vi "Match first tags.vi"(9 "Hyperlink":string, 11 "Text":string) -> (1 "Array":T2(array[cluster]), 3 "Find tag ?":bool)   [LabVIEW 2019, in "Exaprom PDF.lvlib"]
doc: "Version 1.0\nDeveloped by Jean-Marc Simard\nCopyright © 2010, Exaprom Inc.\nAll rights reserved.\nLicense: BSD"
uses:
  Controls/Text Controls/Text type.ctl
  Exaprom PDF.lvlib
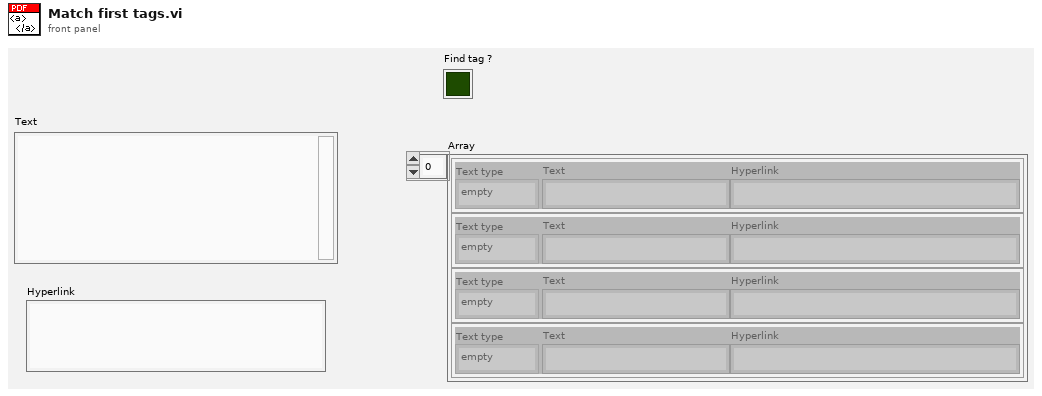
[diagram p1: front panel]
types:
  T1 = typedef "Exaprom PDF.lvlib/Text type.ctl" = enum16{"empty", "Text", "Hyperlink"}
  T2 = cluster{"Text type":T1, "Text":string, "Hyperlink":string}[]
  T3 = cluster{"Text type":T1, "Text type":T1, "Text type":T1}
  T4 = cluster{"Text type":T1, "Text":string, "Hyperlink":string}
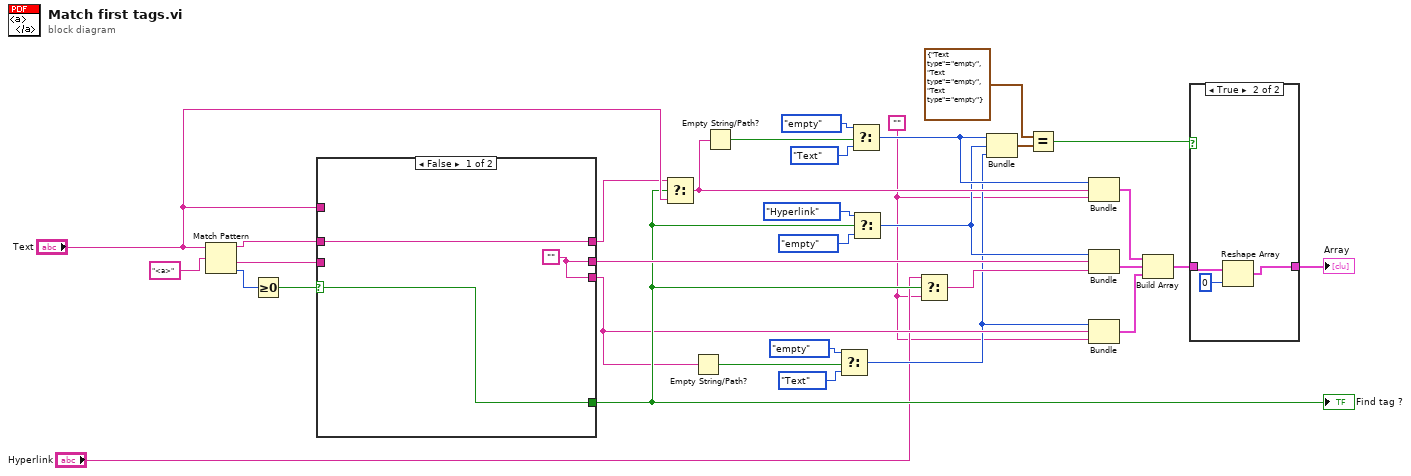
[diagram p0: block diagram]
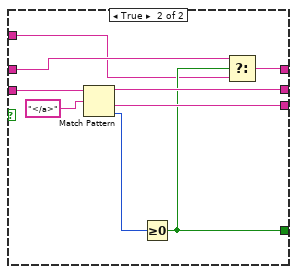
[diagram p3: hidden frame]
diagram:
  w1 = ""
  n1 = Match Pattern(string="Text", regular expression="<a>") -> (before substring=w29:string, after substring=w28:string, offset past match=w32:i32)  [unwired: 2 out]
  n2 = Greater Or Equal To 0?(x=w32) -> (x >= 0?=w31:bool)
  n3 = case shown="False" w31 {
    selector: w31 -> [w34 _]
    tunnel: w29 -> [w36 w38]
    tunnel: [w36 w40] -> w22
    tunnel: w28 -> [_ w45]
    tunnel: [w35 w43] -> w27
    tunnel: [w35 w42] -> w11
    tunnel: [w34 w39] -> w16
    tunnel: "Text" -> [_ w37]
    frame False {
      w35 = ""
    }
    frame True {
      n4 = Match Pattern(string=w45, regular expression="</a>") -> (before substring=w43:string, after substring=w42:string, offset past match=w41:i32)  [unwired: 2 out]
      n5 = Greater Or Equal To 0?(x=w41) -> (x >= 0?=w39:bool)
      n6 = Select(t=w38, s=w39, f=w37) -> (s? t:f=w40:string)
    }
  }
  "Find tag ?" <- w16
  n7 = Select(t=w22, s=w16, f="Text") -> (s? t:f=w15:string)
  n8 = Empty String/Path?(string/path=w11) -> (empty?=w12:bool)
  n9 = Empty String/Path?(string/path=w15) -> (empty?=w21:bool)
  n10 = Select(t=Text_type."empty" ("Text type"), s=w12, f=Text_type."Text" ("Text type")) -> (s? t:f=w8:T1)
  n11 = Select(t=Text_type."empty" ("Text type"), s=w21, f=Text_type."Text" ("Text type")) -> (s? t:f=w10:T1)
  n12 = Select(t=Text_type."Hyperlink" ("Text type"), s=w16, f=Text_type."empty" ("Text type")) -> (s? t:f=w9:T1)
  n13 = Select(t="Hyperlink", s=w16, f=w1) -> (s? t:f=w26:string)
  n14 = Bundle("Text type"=w10, "Text type"=w9, "Text type"=w8) -> (w7:T3)  [unwired: 1 out]
  n15 = Equal?(x=T3 {"Text type"=enum."empty", "Text type"=enum."empty", "Text type"=enum."empty"}, y=w7) -> (x = y?=w5:bool)
  n16 = Bundle("Text type"=w10, "Text"=w15, w1) -> (w25:cluster{"Text type":T1, "Text":string, string})  [unwired: 1 out]
  n17 = Bundle("Text type"=w9, "Text"=w27, "Hyperlink"=w26) -> (w24:T4)  [unwired: 1 out]
  n18 = Bundle("Text type"=w8, "Text"=w11, w1) -> (w23:cluster{"Text type":T1, "Text":string, string})  [unwired: 1 out]
  n19 = Build Array(w25, w24, w23) -> (w4:T2)
  n20 = case shown="True" w5 {
    tunnel: w4 -> [w46 w49]
    tunnel: [w46 w48] -> w3
    frame False {
    }
    frame True {
      n21 = Reshape Array(w49, 0 ("dimension size")) -> (w48:T2)
    }
  }
  "Array" <- w3
